vi "place sensor on baseplate v3.vi"() -> ()   [LabVIEW 2021]
uses:
  Classes/Routine/Routine Enum.ctl
  Classes/Workspace/Fixture Enum.ctl
  Classes/Assembly/Assembly Run.lvclass
  Classes/Controller/Controller.lvclass
  Classes/Routine/Routine.lvclass
  Classes/Workspace/Fixture.lvclass
panel:
  in  "Fixtures":T1[](array[typedef])
  in  "Routine":T2[](array[typedef])
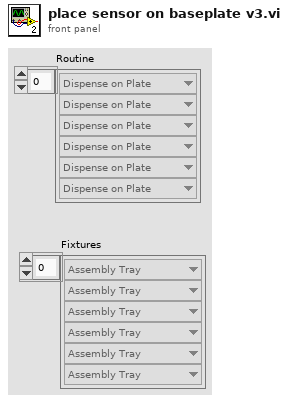
[diagram p1: front panel]
types:
  T1 = typedef "Fixture.lvclass/Fixture Enum.ctl" = enum16{"Assembly Tray", "Syringe Space", "Component", "Pick Up Tool", "Current Position"}
  T2 = typedef "Routine.lvclass/Routine Enum.ctl" = enum16{"Primary Pick Up", "Pick Up All", "Put Down Secondary", "Put Down All", "Release Syringe", "Secondary Pick Up", "Secure Syringe", "Dispense on Plate", "Dispense on Kapton", "Dispense on Sensor"}
  T3 = typedef "Controller.lvclass/Controllers.ctl" = cluster{"I-O.lvclass":refnum<class "I-O.lvclass">, "Gantry":refnum<k24>, "Dispenser":refnum<visa-resource-name>}
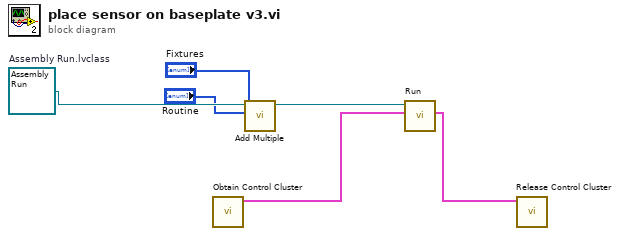
[diagram p0: block diagram]
diagram:
  w6 = refnum<class "Assembly Run.lvclass"> refnum  # Assembly Run.lvclass
  n1 = call "Obtain Control Cluster.vi"() -> ("Control Out"=w2:T3)  [unwired: 11 in]
  n2 = call-dynamic "Add Multiple.vi"("Fixtures"="Fixtures", "Routine"="Routine", "Assembly in"=w6) -> ("Assembly out"=w3:refnum<class "Assembly Run.lvclass">)  [unwired: 7 in, 1 out]
  n3 = call-dynamic "Run.vi"("Control In"=w2, "Assembly In"=w3) -> ("Control Out"=w1:T3)  [unwired: 7 in, 2 out]
  n4 = call "Release Control Cluster.vi"("output cluster"=w1) -> ()  [unwired: 11 in]
